vi "get all by type.vi"(8 "error in (no error)":errorcluster, 10 "Type":refnum<class "system object.lvclass">, 11 "SysObj in":refnum<class "system object.lvclass">) -> (0 "error out":errorcluster, 2 "All objects":refnum<class "system object.lvclass">[](array[class]), 3 "SysObj out":refnum<class "system object.lvclass">)   [LabVIEW 2020, in "system object.lvclass"]
uses:
  system object.lvclass
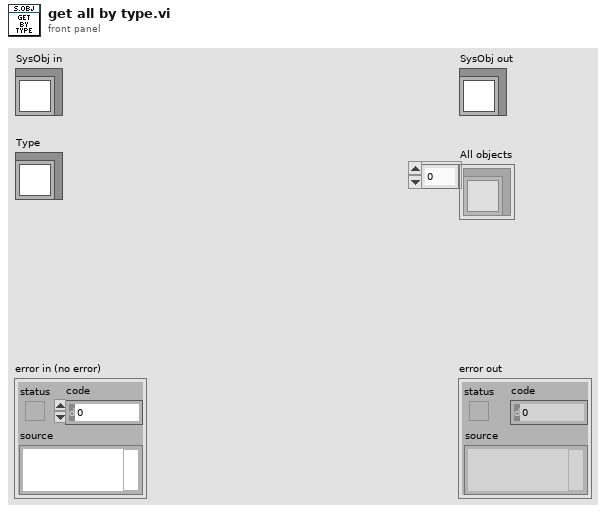
[diagram p1: front panel]
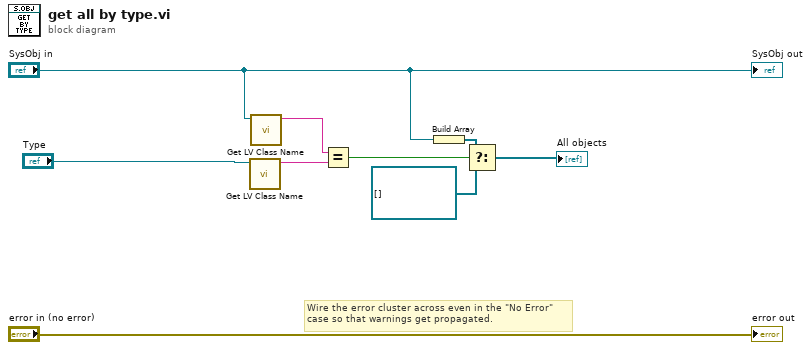
[diagram p0: block diagram]
diagram:
  # "Wire the error cluster across even in the \"No Error\"\ncase so that warnings get propagated."
  n1 = call <vilib>:"Get LV Class Name.vi"("object"="Type") -> ("class name"=w7:string)  [unwired: 9 in, 1 out]
  n2 = call <vilib>:"Get LV Class Name.vi"("object"="SysObj in") -> ("class name"=w6:string)  [unwired: 9 in, 1 out]
  n3 = Equal?(x=w6, y=w7) -> (x = y?=w5:bool)
  n4 = Build Array("SysObj in") -> (w4:refnum<class "system object.lvclass">[])
  n5 = Select(t=w4, s=w5, f=refnum<class "system object.lvclass">[] []) -> (s? t:f=→"All objects":refnum<class "system object.lvclass">[])
  "error out" <- "error in (no error)"
  "SysObj out" <- "SysObj in"
